vi "sub_waveform_to_JSON.vi"() -> ()   [LabVIEW 2013, in "daqio minimal.lvlib"]
uses:
  daqio minimal.lvlib
panel:
  out "error out":errorcluster
  in  "error in (no error)":errorcluster
  out "JSON string":string
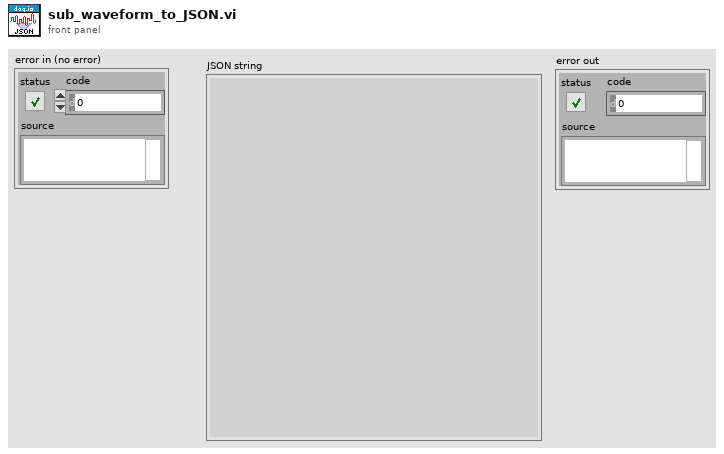
[diagram p1: front panel]
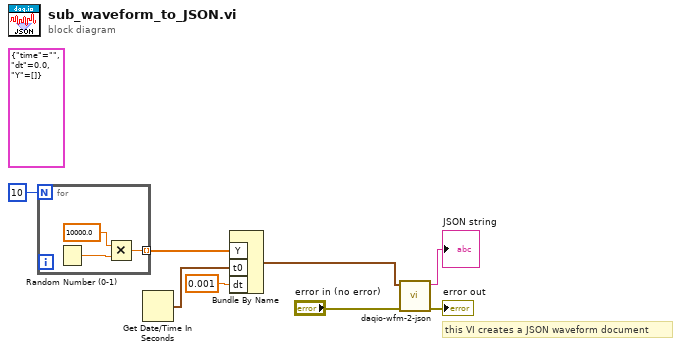
[diagram p0: block diagram]
diagram:
  (unwired) cluster{"time":string, "dt":dbl, "Y":dbl[]} {"time"="", "dt"=0.0, "Y"=[]} ("output cluster")
  # "this VI creates a JSON waveform document"
  n1 = for {
    N: 10 -> [_]
    tunnel: [w10] -> w6 mode=indexing
    n2 = Random Number (0-1)() -> (number: 0 to 1=w11:dbl)
    n3 = Multiply(x=10000.0, y=w11) -> (x*y=w10:dbl)
  }
  n4 = Get Date/Time In Seconds() -> (seconds since 1Jan1904=w3:timestamp)
  n5 = Bundle By Name("Y"=w6, "t0"=w3, "dt"=0.001) -> (w5:waveform(dbl))  [unwired: 1 in]
  n6 = call "daqio-wfm-2-json.vi"("error in (no error)"="error in (no error)", "waveform in"=w5) -> ("error out"=→"error out":errorcluster, "JSON string"=→"JSON string":string)  [unwired: 8 in]
